vi "Teleop_Debugger_02182012.vi"(10 "Match Info":T3={"Autonomous Elapsed Seconds"=0.0, "TeleOp Elapsed Seconds"=0.0, "Disabled Elapsed Seconds"=0.0, "Visited Autonomous"=FALSE, "Visited TeleOp"=FALSE, "Visited Disabled"=FALSE, "Autonomous Settings"={"Autonomous Style"=enum."Independent", "VI Refnum"=refnum}}, 11 "Call Context":T4) -> ()   [LabVIEW 2011]
doc: "This VI is called for each TeleOp packet received from the DS where the robot is not disabled. It is often used to read from the joysticks and update I/O or to update setpoints for timed control loops. It should complete and return within 20 milliseconds or it may miss DS packets."
uses:
  <vilib>/Rock Robotics/WPI/DriverStation/WPI_DriverStationDerivedRobotMode.ctl
  <vilib>/Rock Robotics/WPI/DriverStation/WPI_DriverStationMatch Info.ctl
  <vilib>/Rock Robotics/WPI/Joystick/WPI_JoystickButtonState.ctl
  Robot Global Data.vi
  <vilib>/Rock Robotics/WPI/RobotDrive/WPI_RobotDriveArcadeDrive_Standard(NoSaturation).vi
  <vilib>/Rock Robotics/WPI/DriverStation/DriverStationLCD/WPI_DriverStationLCDLCDLine.ctl
  <vilib>/addons/control/pid/NI_PID_pid.lvlib
  <vilib>/addons/control/pid/pid.llb/PID (DBL).vi
panel:
  out "KINECT_BTNS":T1
  out "LEFT_ARM_AXES":T2
  out "RIGHT_ARM_AXES":T2
  in  "Ball_Sucker_Speed":cluster{"time":dbl, "Arm Pos 1":dbl}[](array[cluster])=[{"time"=2.2540983606557377, "Arm Pos 1"=-0.5639931736228638}] {"Arm Pos 1" scale=1.0..-1.0 scale format="%#_4g"; "time" scale=0.0..5.0}
  in  "Shoot_Feed_Speed":cluster{"time":dbl, "Arm Pos 1":dbl}[](array[cluster])=[{"time"=2.2540983606557377, "Arm Pos 1"=-0.5639931736228638}] {"Arm Pos 1" scale=1.0..-1.0 scale format="%#_4g"; "time" scale=0.0..5.0}
  in  "Shooter_Speed":cluster{"time":dbl, "Arm Pos 1":dbl}[](array[cluster])=[{"time"=2.2540983606557377, "Arm Pos 1"=-0.5639931736228638}] {"Arm Pos 1" scale=1.0..-1.0 scale format="%#_4g"; "time" scale=0.0..5.0}
  in  "REV Lift Limit":dbl(slide)=-0.7802197802197803 scale=1.0..-1.0
  in  "FWD Lift Limit":dbl(slide)=0.7252747252747253 scale=1.0..-1.0
  out "Lift PWR":dbl(slide) scale=-1.0..1.0
  in  "Down Arm Limit":dbl(knob)=0.6049517955629627 scale=1.0..-1.0 scale format="%#_4g"
  in  "UP Arm Limit":dbl(knob)=-0.5066217798191952 scale=1.0..-1.0 scale format="%#_4g"
  out "Arm PWR":dbl(knob) scale=-1.0..1.0
  in  "ShooterAngle3":cluster{"time":dbl, "Arm Pos 1":dbl}[](array[cluster])=[{"time"=2.2540983606557377, "Arm Pos 1"=-0.5639931736228638}] {"Arm Pos 1" scale=1.0..-1.0 scale format="%#_4g"; "time" scale=0.0..5.0}
  in  "ShooterAngle2":cluster{"time":dbl, "Arm Pos 1":dbl}[](array[cluster])=[{"time"=2.2540983606557377, "Arm Pos 1"=-0.5639931736228638}] {"Arm Pos 1" scale=1.0..-1.0 scale format="%#_4g"; "time" scale=0.0..5.0}
  in  "ShooterAngle1":cluster{"time":dbl, "Arm Pos 1":dbl}[](array[cluster])=[{"time"=2.2540983606557377, "Arm Pos 1"=-0.5639931736228638}] {"Arm Pos 1" scale=1.0..-1.0 scale format="%#_4g"; "time" scale=0.0..5.0}
  in  "Boost_Rate":dbl=1.5
  out "JS1_BTNS":T1
  out "JS1_AXES":T2
  out "JS2_BTNS":T1
  out "JS2_AXES":T2
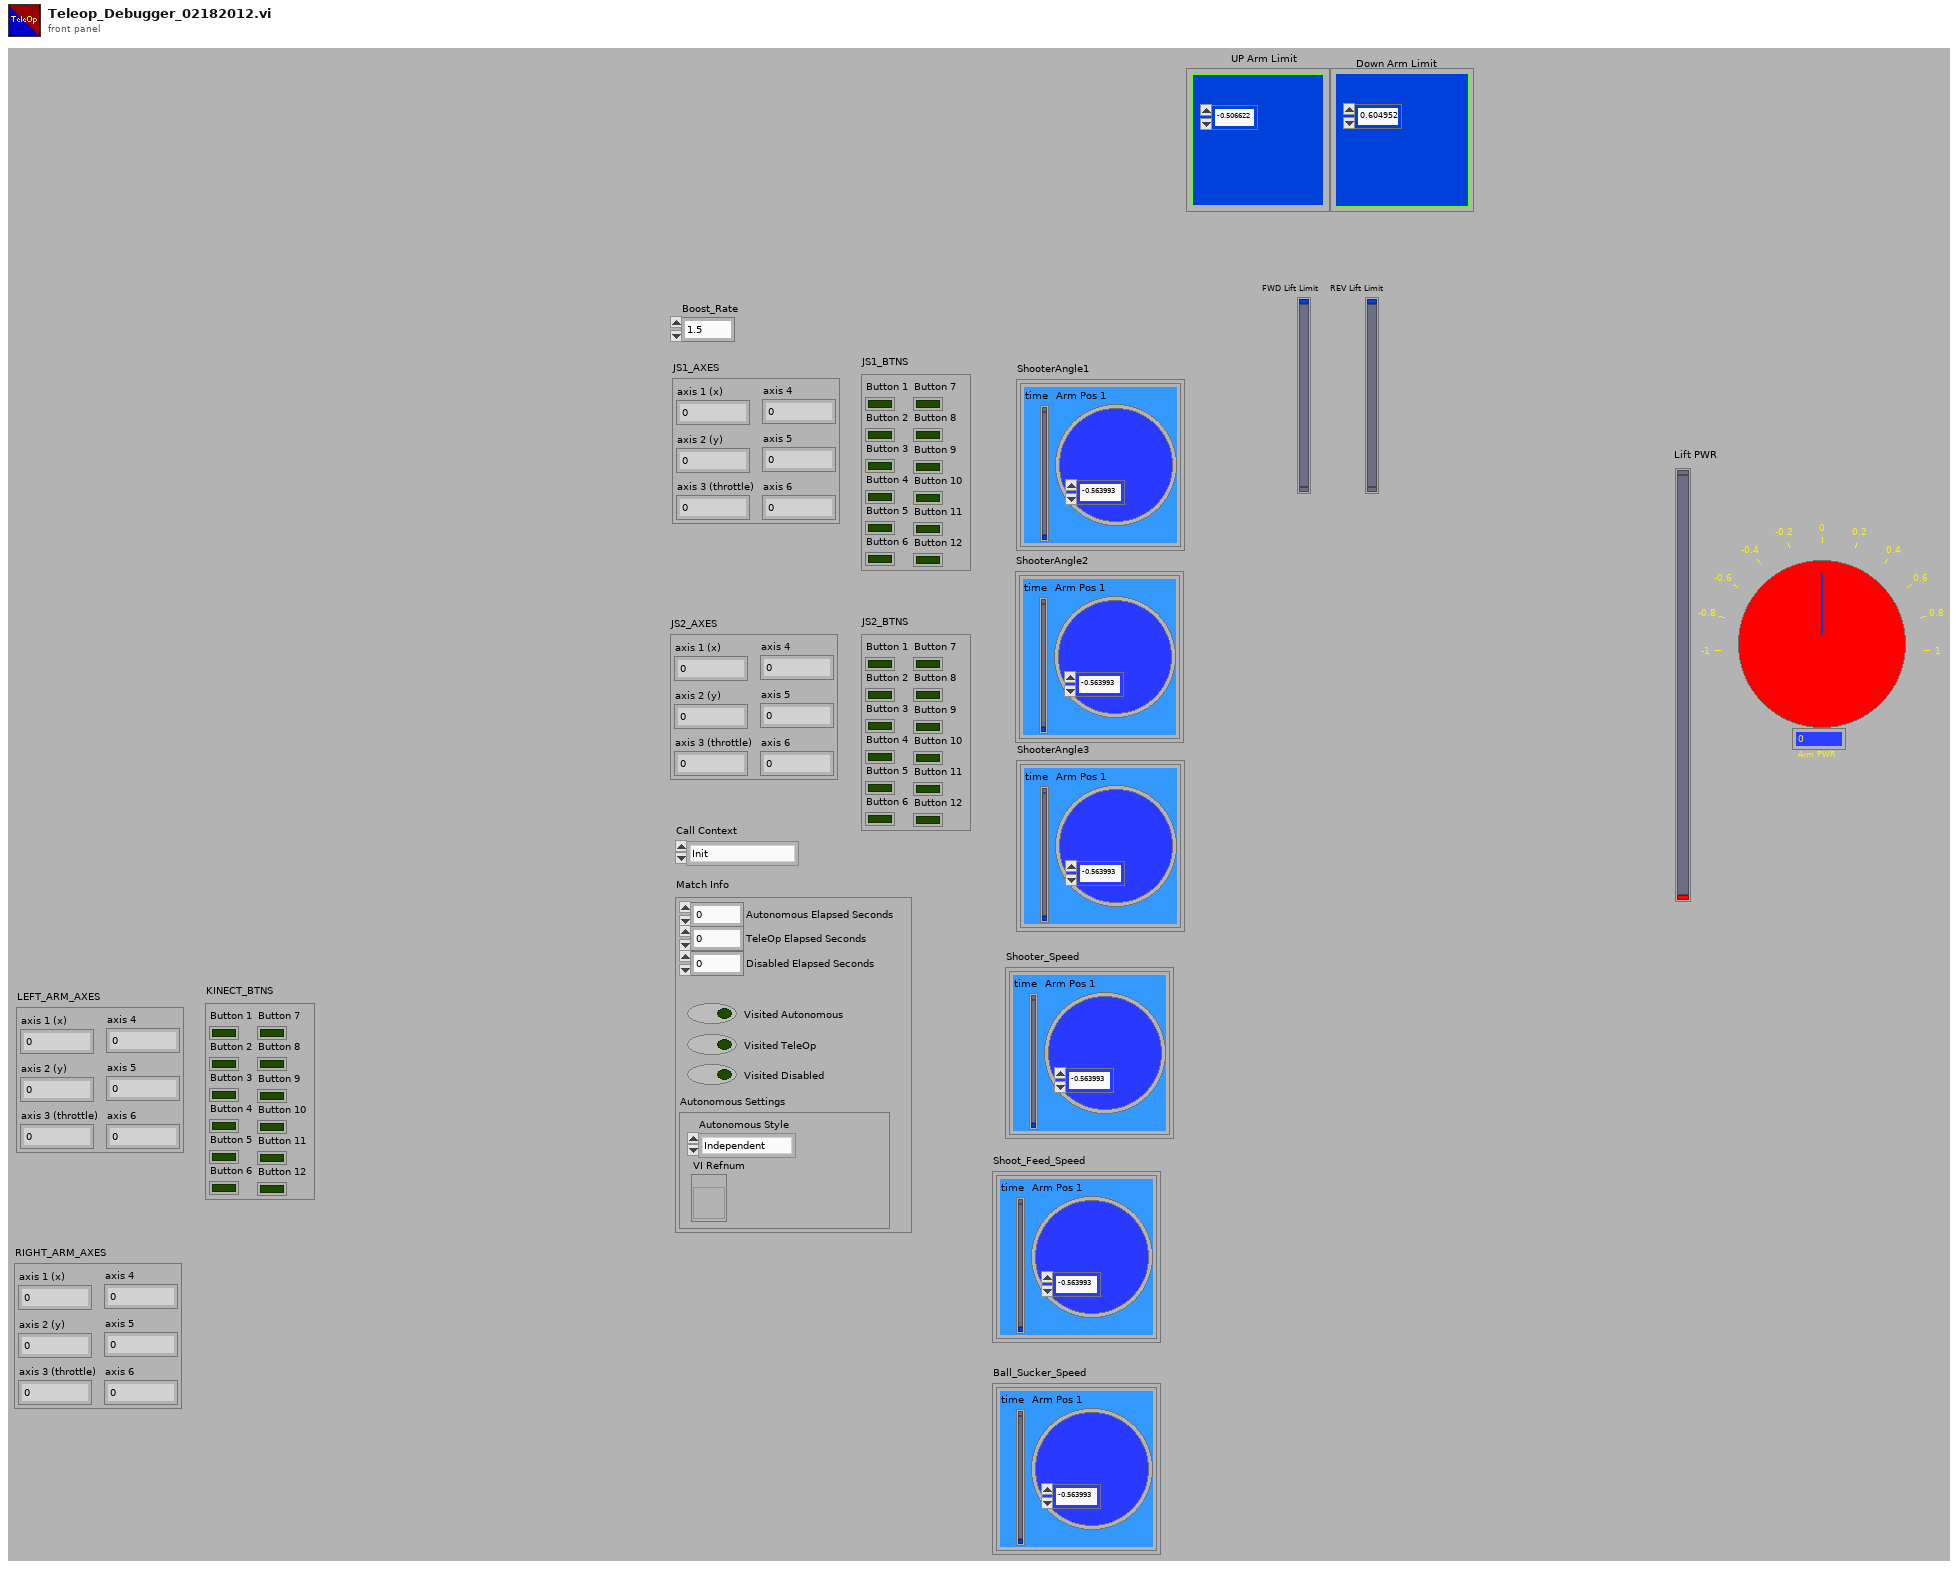
[diagram p1: front panel]
types:
  T1 = typedef "WPI_JoystickButtonState.ctl" = cluster{"Button 1":bool, "Button 2":bool, "Button 3":bool, "Button 4":bool, "Button 5":bool, "Button 6":bool, "Button 7":bool, "Button 8":bool, "Button 9":bool, "Button 10":bool, "Button 11":bool, "Button 12":bool}
  T2 = cluster{"axis 1 (x)":dbl, "axis 2 (y)":dbl, "axis 3 (throttle)":dbl, "axis 4":dbl, "axis 5":dbl, "axis 6":dbl}
  T3 = typedef "WPI_DriverStationMatch Info.ctl" = cluster{"Autonomous Elapsed Seconds":dbl, "TeleOp Elapsed Seconds":dbl, "Disabled Elapsed Seconds":dbl, "Visited Autonomous":bool, "Visited TeleOp":bool, "Visited Disabled":bool, "Autonomous Settings":cluster{"Autonomous Style":enum16{"Iterative", "Independent"}, "VI Refnum":refnum<vi>}}
  T4 = typedef "WPI_DriverStationDerivedRobotMode.ctl" = enum16{"Init", "Execute", "Stop"}
  T5 = typedef "WPI_JoystickDevRef.ctl" = cluster{"Device":T6}
  T6 = typedef "WPI_JoystickDeviceEnum.ctl" = enum16{"USB 1", "USB 2", "USB 3", "USB 4", "Kinect 1", "Kinect 2"}
  T7 = typedef "WPI_MotorControlDeviceRef.ctl" = cluster{"DeviceStatus":errorcluster, "Type":enum16{"PWM", "CAN"}, "PWM":cluster{"Digital Module":T8, "PWM Channel":T9, "DeadBand":T10}, "CAN":cluster{"Device Number":u8, "Control Mode":T11, "Semaphore":T12, "Max Vout":dbl}, "Invert":bool, "TransformRef":T13, "InvTransformRef":T13}
  T8 = typedef "FPGA_TypedefDigitalModule.ctl" = enum16{"Digital Module 1", "Digital Module 2"}
  T9 = typedef "FPGA_DIOPWMChannel.ctl" = enum8{"PWM 1", "PWM 2", "PWM 3", "PWM 4", "PWM 5", "PWM 6", "PWM 7", "PWM 8", "PWM 9", "PWM 10", "Invalid"}
  T10 = typedef "WPI_PWMDeadband.ctl" = cluster{"Name":string, "maxPositivePwm":i32, "minPositivePwm":i32, "centerPwm":i32, "maxNegativePwm":i32, "minNegativePwm":i32, "angularRange":u16}
  T11 = typedef "WPI_CANJaguar_ControlMode.ctl" = enum8{"Percent VBus", "Current", "Speed", "Position", "Voltage"}
  T12 = typedef "Semaphore RefNum" = refnum<k1>
  T13 = typedef "WPI_PWMTransform_ConPane.ctl" = refnum<vi>
  T14 = typedef "WPI_DriverStationLCDLCDLine.ctl" = enum16{"Main - Line 1", "User - Line 2", "User - Line 3", "User - Line 4", "User - Line 5", "User - Line 6"}
  T15 = typedef "WPI_ServoDeviceRef.ctl" = cluster{"DeviceStatus":errorcluster, "Digital Module":T8, "PWM Channel":T9, "DeadBand":T10}
  T16 = typedef "WPI_RobotDriveDevRef.ctl" = cluster{"DevStatus":errorcluster, "Motors[]":T7[], "Square Inputs":bool, "Max Output":dbl, "Isochronous":bool}
  T17 = cluster{"proportional gain (Kc)":dbl, "integral time (Ti, min)":dbl, "derivative time (Td, min)":dbl}
  T18 = typedef "WPI_AnalogChannelDevRef.ctl" = cluster{"DevStatus":errorcluster, "Analog Module":T19, "Analog Channel":T20}
  T19 = typedef "FPGA_TypedefAnalogModule.ctl" = enum16{"Analog Module 1", "Analog Module 2"}
  T20 = typedef "FPGA_AIChannel.ctl" = enum8{"AI 1", "AI 2", "AI 3", "AI 4", "AI 5", "AI 6", "AI 7", "AI 8", "Invalid"}
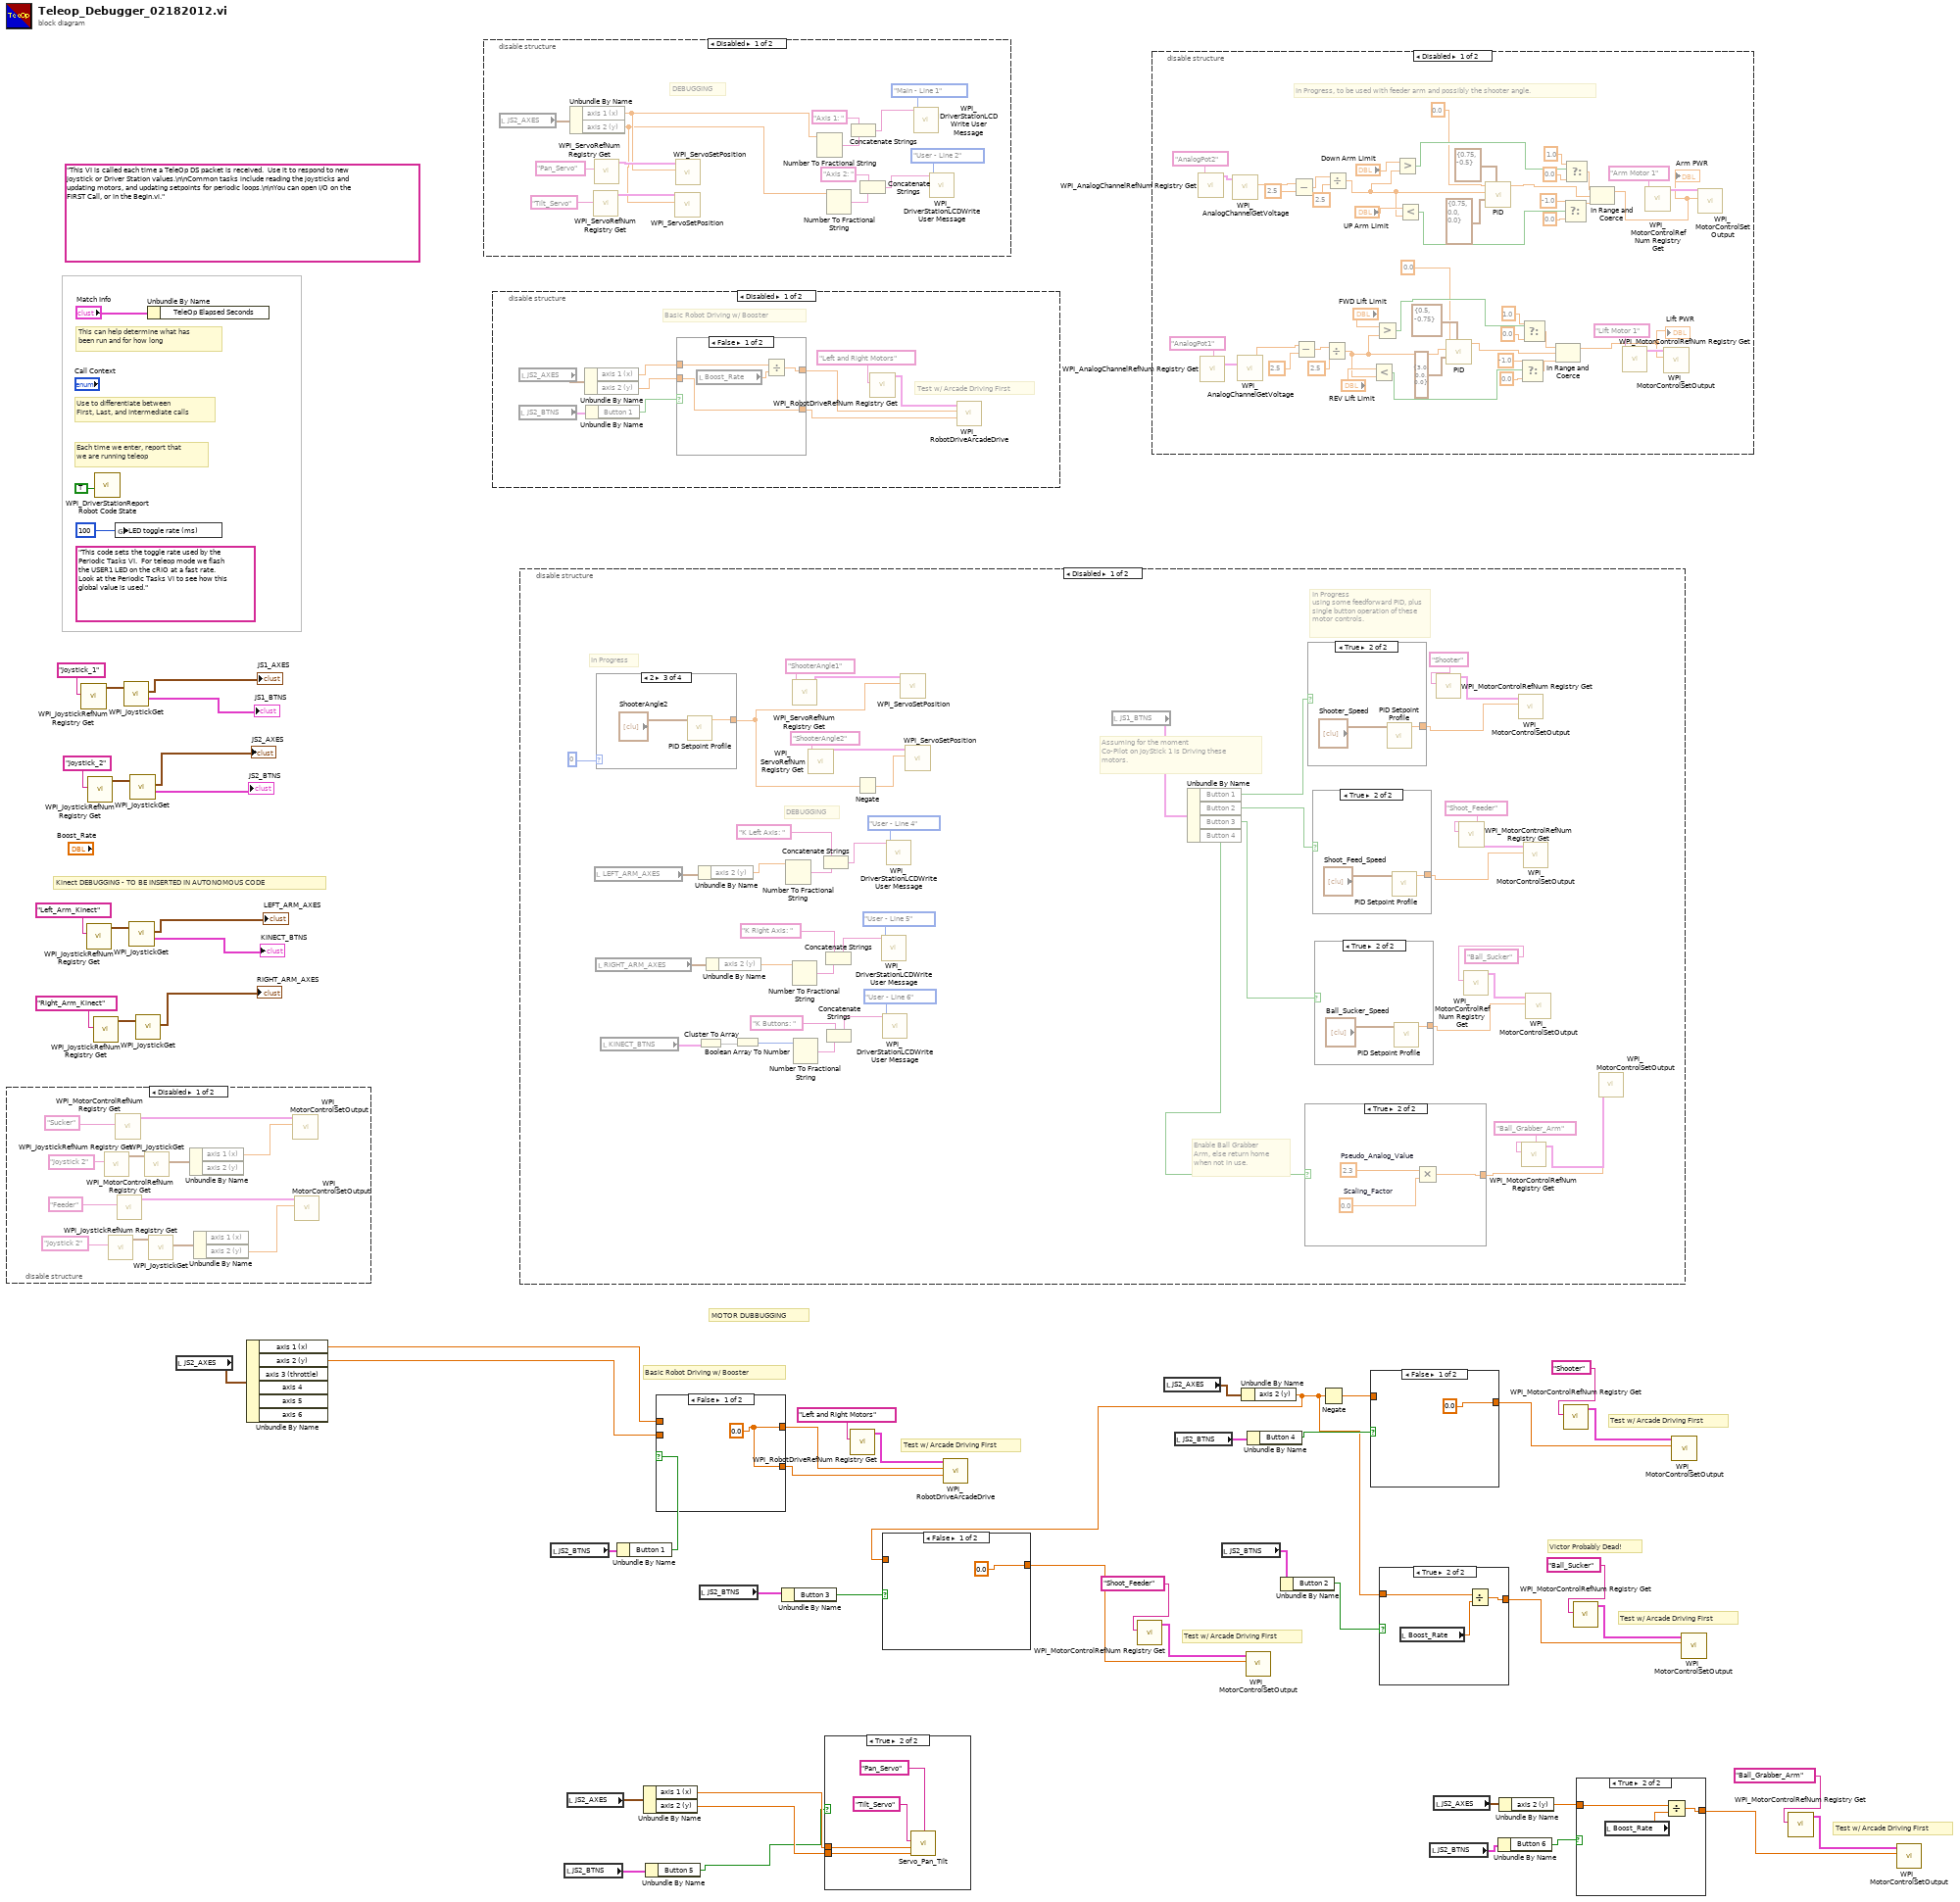
[diagram p0: block diagram]
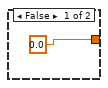
[diagram p3: hidden frame]
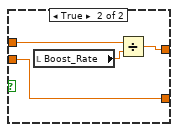
[diagram p4: hidden frame]
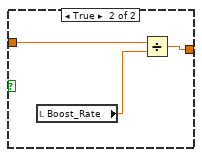
[diagram p5: hidden frame]
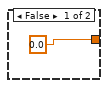
[diagram p6: hidden frame]
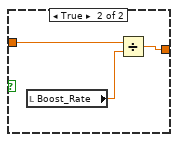
[diagram p7: hidden frame]
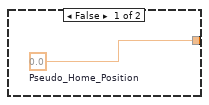
[diagram p10: hidden frame]
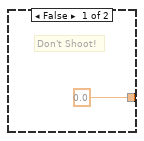
[diagram p11: hidden frame]
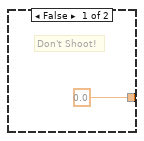
[diagram p12: hidden frame]
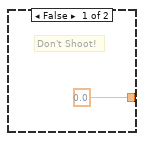
[diagram p13: hidden frame]
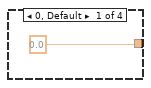
[diagram p14: hidden frame]
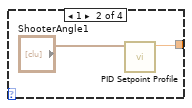
[diagram p15: hidden frame]
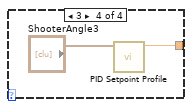
[diagram p16: hidden frame]
diagram:
  (unwired) "This code sets the toggle rate used by the Periodic Tasks VI.  For teleop mode we flash the USER1 LED on the cRIO at a fast rate.  Look at the Periodic Tasks VI to see how this global value is used."
  (unwired) "This VI is called each time a TeleOp DS packet is received.  Use it to respond to new joystick or Driver Station values.\n\nCommon tasks include reading the joysticks and updating motors, and updating setpoints for periodic loops.\n\nYou can open I/O on the FIRST Call, or in the Begin.vi."
  # "Victor Probably Dead!"
  # "Test w/ Arcade Driving First"
  # "Basic Robot Driving w/ Booster"
  # "Test w/ Arcade Driving First"
  # "Test w/ Arcade Driving First"
  # "Test w/ Arcade Driving First"
  # "Test w/ Arcade Driving First"
  # "MOTOR DUBBUGGING"
  # "Kinect DEBUGGING - TO BE INSERTED IN AUTONOMOUS CODE"
  # "Each time we enter, report that\nwe are running teleop"
  # "Use to differentiate between\nFirst, Last, and Intermediate calls"
  # "This can help determine what has\nbeen run and for how long"
  n1 = disable-structure shown="Disabled" {
    frame Disabled {
      n2 = call <vilib>:"WPI_JoystickRefNum Registry Get.vi"("refnum name"="Joystick 2") -> ("JoystickDevRef"=w67:T5)  [unwired: 1 in, 9 out]
      n3 = call <vilib>:"WPI_JoystickRefNum Registry Get.vi"("refnum name"="Joystick 2") -> ("JoystickDevRef"=w61:T5)  [unwired: 1 in, 9 out]
      n4 = call <vilib>:"WPI_MotorControlRefNum Registry Get.vi"("refnum name"="Sucker") -> ("MotorControlDevRef"=w66:T7)  [unwired: 9 in, 1 out]
      n5 = call <vilib>:"WPI_MotorControlRefNum Registry Get.vi"("refnum name"="Feeder") -> ("MotorControlDevRef"=w60:T7)  [unwired: 9 in, 1 out]
      n6 = call <vilib>:"WPI_JoystickGet.vi"("JoystickDevRef"=w67) -> ("Axes"=w69:T2)  [unwired: 1 in, 5 out]
      n7 = call <vilib>:"WPI_JoystickGet.vi"("JoystickDevRef"=w61) -> ("Axes"=w63:T2)  [unwired: 1 in, 5 out]
      n8 = Unbundle By Name(w69) -> ("axis 1 (x)"=w64:dbl)  [unwired: 1 out]
      n9 = Unbundle By Name(w63) -> ("axis 2 (y)"=w58:dbl)  [unwired: 1 out]
      n10 = call <vilib>:"WPI_MotorControlSetOutput.vi"("Output"=w64, "MotorControlDevRef"=w66) -> ()  [unwired: 8 in, 2 out]
      n11 = call <vilib>:"WPI_MotorControlSetOutput.vi"("Output"=w58, "MotorControlDevRef"=w60) -> ()  [unwired: 8 in, 2 out]
    }
    frame Enabled {
    }
  }
  n12 = call <vilib>:"WPI_JoystickRefNum Registry Get.vi"("refnum name"="Joystick_1") -> ("JoystickDevRef"=w50:T5)  [unwired: 1 in, 9 out]
  n13 = call <vilib>:"WPI_JoystickRefNum Registry Get.vi"("refnum name"="Left_Arm_Kinect") -> ("JoystickDevRef"=w43:T5)  [unwired: 1 in, 9 out]
  n14 = call <vilib>:"WPI_JoystickRefNum Registry Get.vi"("refnum name"="Joystick_2") -> ("JoystickDevRef"=w52:T5)  [unwired: 1 in, 9 out]
  n15 = call <vilib>:"WPI_JoystickRefNum Registry Get.vi"("refnum name"="Right_Arm_Kinect") -> ("JoystickDevRef"=w45:T5)  [unwired: 1 in, 9 out]
  n16 = call <vilib>:"WPI_DriverStationReport Robot Code State.vi"("TeleOp"=TRUE ("Autonomous")) -> ()  [unwired: 10 in, 1 out]
  n17 = global write "Robot Global Data.vi" "LED toggle rate (ms)"(u32 100 ("LED ms toggle rate")) -> ()
  n18 = call <vilib>:"WPI_JoystickGet.vi"("JoystickDevRef"=w50) -> ("Buttons"=→"JS1_BTNS":T1, "Axes"=→"JS1_AXES":T2)  [unwired: 1 in, 4 out]
  n19 = call <vilib>:"WPI_JoystickGet.vi"("JoystickDevRef"=w43) -> ("Buttons"=→"KINECT_BTNS":T1, "Axes"=→"LEFT_ARM_AXES":T2)  [unwired: 1 in, 4 out]
  n20 = call <vilib>:"WPI_JoystickGet.vi"("JoystickDevRef"=w52) -> ("Buttons"=→"JS2_BTNS":T1, "Axes"=→"JS2_AXES":T2)  [unwired: 1 in, 4 out]
  n21 = call <vilib>:"WPI_JoystickGet.vi"("JoystickDevRef"=w45) -> ("Axes"=→"RIGHT_ARM_AXES":T2)  [unwired: 1 in, 5 out]
  n22 = Unbundle By Name("Match Info") -> ()  [unwired: 1 out]
  n23 = local read "JS2_AXES"() -> (w25:T2)
  n24 = Unbundle By Name(w25) -> ("axis 1 (x)"=w21:dbl, "axis 2 (y)"=w20:dbl)  [unwired: 4 out]
  n25 = disable-structure shown="Disabled" {
    frame Disabled {
      # "DEBUGGING"
      n26 = local read "JS2_AXES"() -> (w70:T2)
      n27 = Unbundle By Name(w70) -> ("axis 1 (x)"=w72:dbl, "axis 2 (y)"=w71:dbl)
      n28 = call <vilib>:"WPI_ServoRefNum Registry Get.vi"("refnum name"="Tilt_Servo") -> ("ServoDeviceRef"=w83:T15)  [unwired: 9 in, 1 out]
      n29 = call <vilib>:"WPI_ServoRefNum Registry Get.vi"("refnum name"="Pan_Servo") -> ("ServoDeviceRef"=w81:T15)  [unwired: 9 in, 1 out]
      n30 = call <vilib>:"WPI_ServoSetPosition.vi"("Position"=w71, "ServoDeviceRef"=w83) -> ()  [unwired: 8 in, 2 out]
      n31 = call <vilib>:"WPI_ServoSetPosition.vi"("Position"=w72, "ServoDeviceRef"=w81) -> ()  [unwired: 8 in, 2 out]
      n32 = Number To Fractional String(number=w72) -> (F-format string=w78:string)  [unwired: 3 in]
      n33 = Number To Fractional String(number=w71) -> (F-format string=w76:string)  [unwired: 3 in]
      n34 = Concatenate Strings("Axis 1: ", w78) -> (w75:string)
      n35 = Concatenate Strings("Axis 2: ", w76) -> (w73:string)
      n36 = call <vilib>:"WPI_DriverStationLCDWrite User Message.vi"("line text"=w75, "line"=WPI_DriverStationLCDLCDLine."Main - Line 1") -> ()  [unwired: 13 in, 1 out]
      n37 = call <vilib>:"WPI_DriverStationLCDWrite User Message.vi"("line text"=w73, "line"=WPI_DriverStationLCDLCDLine."User - Line 2") -> ()  [unwired: 13 in, 1 out]
    }
    frame Enabled {
    }
  }
  n38 = disable-structure shown="Disabled" {
    frame Disabled {
      # "Basic Robot Driving w/ Booster"
      # "Test w/ Arcade Driving First"
      n39 = local read "JS2_BTNS"() -> (w90:T1)
      n40 = local read "JS2_AXES"() -> (w91:T2)
      n41 = Unbundle By Name(w91) -> ("axis 1 (x)"=w87:dbl, "axis 2 (y)"=w86:dbl)
      n42 = Unbundle By Name(w90) -> ("Button 1"=w85:bool)
      n43 = case shown="False" w85 {
        tunnel: w86 -> [w94 w98]
        tunnel: [w94 w98] -> w88
        tunnel: w87 -> [w97 w99]
        tunnel: [w96 w99] -> w89
        frame False {
          n44 = local read "Boost_Rate"() -> (w95:dbl)
          n45 = Divide(x=w97, y=w95) -> (x/y=w96:dbl)
        }
        frame True {
        }
      }
      n46 = call <vilib>:"WPI_RobotDriveRefNum Registry Get.vi"("refnum name"="Left and Right Motors") -> ("RobotDriveDevRef"=w92:T16)  [unwired: 1 in, 9 out]
      n47 = call-poly <vilib>:"WPI_RobotDriveArcadeDrive.vi"("Y axis value"=w88, "X axis value"=w89, "RobotDriveDevRef"=w92) -> ()  [unwired: 7 in, 2 out]
    }
    frame Enabled {
    }
  }
  n48 = disable-structure shown="Disabled" {
    frame Disabled {
      # "DEBUGGING"
      # "Enable Ball Grabber\nArm, else return home\nwhen not in use."
      # "Assuming for the moment\nCo-Pilot on JoyStick 1 is Driving these\nmotors."
      # "In Progress\nusing some feedforward PID, plus\nsingle button operation of these \nmotor controls."
      # "In Progress"
      n49 = local read "LEFT_ARM_AXES"() -> (w110:T2)
      n50 = local read "RIGHT_ARM_AXES"() -> (w107:T2)
      n51 = case shown="2" 0 {
        tunnel: [0.0 w157 w159 w161] -> w137
        frame 0, Default {
        }
        frame 1 {
          n52 = call <vilib>:"PID Setpoint Profile.vi"("setpoint profile"="ShooterAngle1") -> ("setpoint"=w157:dbl)  [unwired: 2 in, 6 out]
        }
        frame 2 {
          n53 = call <vilib>:"PID Setpoint Profile.vi"("setpoint profile"="ShooterAngle2") -> ("setpoint"=w159:dbl)  [unwired: 2 in, 6 out]
        }
        frame 3 {
          n54 = call <vilib>:"PID Setpoint Profile.vi"("setpoint profile"="ShooterAngle3") -> ("setpoint"=w161:dbl)  [unwired: 2 in, 6 out]
        }
      }
      n55 = local read "KINECT_BTNS"() -> (w102:T1)
      n56 = Unbundle By Name(w110) -> ("axis 2 (y)"=w109:dbl)
      n57 = Cluster To Array(cluster=w102) -> (array=w101:bool[])
      n58 = Unbundle By Name(w107) -> ("axis 2 (y)"=w108:dbl)
      n59 = Boolean Array To Number(Boolean array=w101) -> (number=w100:u32)
      n60 = Number To Fractional String(number=w109) -> (F-format string=w116:string)  [unwired: 3 in]
      n61 = call <vilib>:"WPI_ServoRefNum Registry Get.vi"("refnum name"="ShooterAngle1") -> ("ServoDeviceRef"=w141:T15)  [unwired: 1 in, 9 out]
      n62 = Number To Fractional String(number=w108) -> (F-format string=w114:string)  [unwired: 3 in]
      n63 = Number To Fractional String(number=w100) -> (F-format string=w105:string)  [unwired: 3 in]
      n64 = call <vilib>:"WPI_ServoRefNum Registry Get.vi"("refnum name"="ShooterAngle2") -> ("ServoDeviceRef"=w139:T15)  [unwired: 1 in, 9 out]
      n65 = Concatenate Strings("K Left Axis: ", w116) -> (w113:string)
      n66 = Concatenate Strings("K Right Axis: ", w114) -> (w111:string)
      n67 = Concatenate Strings("K Buttons: ", w105) -> (w103:string)
      n68 = Negate(x=w137) -> (-x=w138:dbl)
      n69 = call <vilib>:"WPI_DriverStationLCDWrite User Message.vi"("line text"=w111, "line"=WPI_DriverStationLCDLCDLine."User - Line 5") -> ()  [unwired: 13 in, 1 out]
      n70 = call <vilib>:"WPI_DriverStationLCDWrite User Message.vi"("line text"=w103, "line"=WPI_DriverStationLCDLCDLine."User - Line 6") -> ()  [unwired: 13 in, 1 out]
      n71 = call <vilib>:"WPI_DriverStationLCDWrite User Message.vi"("line text"=w113, "line"=WPI_DriverStationLCDLCDLine."User - Line 4") -> ()  [unwired: 13 in, 1 out]
      n72 = call <vilib>:"WPI_ServoSetPosition.vi"("Position"=w137, "ServoDeviceRef"=w141) -> ()  [unwired: 1 in, 9 out]
      n73 = call <vilib>:"WPI_ServoSetPosition.vi"("Position"=w138, "ServoDeviceRef"=w139) -> ()  [unwired: 1 in, 9 out]
      n74 = local read "JS1_BTNS"() -> (w126:T1)
      n75 = Unbundle By Name(w126) -> ("Button 1"=w125:bool, "Button 2"=w124:bool, "Button 3"=w123:bool, "Button 4"=w120:bool)
      n76 = case shown="True" w120 {
        tunnel: [w143 w144] -> w119
        frame False {
          w143 = 0.0  # Pseudo_Home_Position
        }
        frame True {
          w145 = 0.0  # Scaling_Factor
          w146 = 2.3  # Pseudo_Analog_Value
          n77 = Multiply(x=w146, y=w145) -> (x*y=w144:dbl)
        }
      }
      n78 = case shown="True" w125 {
        tunnel: [0.0 w154] -> w134
        frame False {
          # "Don't Shoot!"
        }
        frame True {
          n79 = call <vilib>:"PID Setpoint Profile.vi"("setpoint profile"="Shooter_Speed") -> ("setpoint"=w154:dbl)  [unwired: 2 in, 6 out]
        }
      }
      n80 = case shown="True" w124 {
        tunnel: [0.0 w151] -> w131
        frame False {
          # "Don't Shoot!"
        }
        frame True {
          n81 = call <vilib>:"PID Setpoint Profile.vi"("setpoint profile"="Shoot_Feed_Speed") -> ("setpoint"=w151:dbl)  [unwired: 2 in, 6 out]
        }
      }
      n82 = case shown="True" w123 {
        tunnel: [0.0 w148] -> w128
        frame False {
          # "Don't Shoot!"
        }
        frame True {
          n83 = call <vilib>:"PID Setpoint Profile.vi"("setpoint profile"="Ball_Sucker_Speed") -> ("setpoint"=w148:dbl)  [unwired: 2 in, 6 out]
        }
      }
      n84 = call <vilib>:"WPI_MotorControlRefNum Registry Get.vi"("refnum name"="Shooter") -> ("MotorControlDevRef"=w133:T7)  [unwired: 9 in, 1 out]
      n85 = call <vilib>:"WPI_MotorControlRefNum Registry Get.vi"("refnum name"="Shoot_Feeder") -> ("MotorControlDevRef"=w130:T7)  [unwired: 9 in, 1 out]
      n86 = call <vilib>:"WPI_MotorControlRefNum Registry Get.vi"("refnum name"="Ball_Sucker") -> ("MotorControlDevRef"=w127:T7)  [unwired: 9 in, 1 out]
      n87 = call <vilib>:"WPI_MotorControlSetOutput.vi"("Output"=w134, "MotorControlDevRef"=w133) -> ()  [unwired: 8 in, 2 out]
      n88 = call <vilib>:"WPI_MotorControlRefNum Registry Get.vi"("refnum name"="Ball_Grabber_Arm") -> ("MotorControlDevRef"=w122:T7)  [unwired: 9 in, 1 out]
      n89 = call <vilib>:"WPI_MotorControlSetOutput.vi"("Output"=w131, "MotorControlDevRef"=w130) -> ()  [unwired: 8 in, 2 out]
      n90 = call <vilib>:"WPI_MotorControlSetOutput.vi"("Output"=w128, "MotorControlDevRef"=w127) -> ()  [unwired: 8 in, 2 out]
      n91 = call <vilib>:"WPI_MotorControlSetOutput.vi"("Output"=w119, "MotorControlDevRef"=w122) -> ()  [unwired: 8 in, 2 out]
    }
    frame Enabled {
    }
  }
  n92 = local read "JS2_BTNS"() -> (w24:T1)
  n93 = local read "JS2_BTNS"() -> (w14:T1)
  n94 = local read "JS2_AXES"() -> (w13:T2)
  n95 = Unbundle By Name(w24) -> ("Button 1"=w19:bool)
  n96 = Unbundle By Name(w13) -> ("axis 1 (x)"=w3:dbl, "axis 2 (y)"=w2:dbl)
  n97 = Unbundle By Name(w14) -> ("Button 5"=w1:bool)
  n98 = case shown="False" w19 {
    tunnel: w20 -> [_ w164]
    tunnel: [w163 w164] -> w22
    tunnel: w21 -> [_ w167]
    tunnel: [w163 w166] -> w23
    frame False {
      w163 = 0.0
    }
    frame True {
      n99 = local read "Boost_Rate"() -> (w165:dbl)
      n100 = Divide(x=w167, y=w165) -> (x/y=w166:dbl)
    }
  }
  n101 = local read "JS2_BTNS"() -> (w18:T1)
  n102 = Unbundle By Name(w18) -> ("Button 3"=w17:bool)
  n103 = case shown="True" w1 {
    tunnel: w3 -> [_ w169]
    tunnel: w2 -> [_ w168]
    frame False {
    }
    frame True {
      n104 = call "Servo_Pan_Tilt.vi"("Tilt_Servo_Position"=w168, "Pan_Servo_Position"=w169, "Tilt_Servo_Name"="Tilt_Servo", "Pan_Servo_Name"="Pan_Servo") -> ()
    }
  }
  n105 = call <vilib>:"WPI_RobotDriveRefNum Registry Get.vi"("refnum name"="Left and Right Motors") -> ("RobotDriveDevRef"=w26:T16)  [unwired: 1 in, 9 out]
  n106 = call-poly <vilib>:"WPI_RobotDriveArcadeDrive.vi"("Y axis value"=w22, "X axis value"=w23, "RobotDriveDevRef"=w26) -> ()  [unwired: 7 in, 2 out]
  n107 = call <vilib>:"WPI_MotorControlRefNum Registry Get.vi"("refnum name"="Shoot_Feeder") -> ("MotorControlDevRef"=w30:T7)  [unwired: 9 in, 1 out]
  n108 = disable-structure shown="Disabled" {
    frame Disabled {
      # "In Progress, to be used with feeder arm and possibly the shooter angle."
      n109 = call <vilib>:"WPI_AnalogChannelRefNum Registry Get.vi"("refnum name"="AnalogPot2") -> ("AIDeviceRef"=w216:T18)  [unwired: 1 in, 9 out]
      n110 = call <vilib>:"WPI_AnalogChannelRefNum Registry Get.vi"("refnum name"="AnalogPot1") -> ("AIDeviceRef"=w193:T18)  [unwired: 1 in, 9 out]
      n111 = call <vilib>:"WPI_AnalogChannelGetVoltage.vi"("AIDeviceRef"=w216) -> ("Voltage"=w212:dbl)  [unwired: 1 in, 9 out]
      n112 = call <vilib>:"WPI_AnalogChannelGetVoltage.vi"("AIDeviceRef"=w193) -> ("Voltage"=w190:dbl)  [unwired: 1 in, 9 out]
      n113 = Subtract(x=w212, y=2.5) -> (x-y=w210:dbl)
      n114 = Subtract(x=w190, y=2.5) -> (x-y=w188:dbl)
      n115 = Divide(x=w188, y=2.5) -> (x/y=w176:dbl)
      n116 = Divide(x=w210, y=2.5) -> (x/y=w198:dbl)
      n117 = Less?(x="REV Lift Limit", y=w176) -> (x < y?=w185:bool)
      n118 = Greater?(x="FWD Lift Limit", y=w176) -> (0:w183:bool)
      n119 = Greater?(x="Down Arm Limit", y=w198) -> (0:w201:bool)
      n120 = Less?(x="UP Arm Limit", y=w198) -> (x < y?=w200:bool)
      n121 = call-poly <vilib>:"PID.vi"("output range"=cluster{"output high":dbl, "output low":dbl} {"output high"=0.5, "output low"=-0.75}, "PID gains"=T17 {"proportional gain (Kc)"=3.0, "integral time (Ti, min)"=0.0, "derivative time (Td, min)"=0.0}, "process variable"=w176, "setpoint"=0.0) -> ("output"=w175:dbl)  [unwired: 2 in, 5 out]
      n122 = call-poly <vilib>:"PID.vi"("output range"=cluster{"output high":dbl, "output low":dbl} {"output high"=0.75, "output low"=-0.5}, "PID gains"=T17 {"proportional gain (Kc)"=0.75, "integral time (Ti, min)"=0.0, "derivative time (Td, min)"=0.0}, "process variable"=w198, "setpoint"=0.0) -> ("output"=w199:dbl)  [unwired: 2 in, 5 out]
      n123 = Select(t=-1.0, s=w185, f=0.0) -> (s? t:f=w182:dbl)
      n124 = Select(t=1.0, s=w183, f=0.0) -> (s? t:f=w181:dbl)
      n125 = In Range and Coerce(upper limit=w181, x=w175, lower limit=w182) -> (coerced(x)=w174:dbl)  [unwired: 1 out]
      "Lift PWR" <- w174
      n126 = Select(t=-1.0, s=w200, f=0.0) -> (s? t:f=w202:dbl)
      n127 = Select(t=1.0, s=w201, f=0.0) -> (s? t:f=w203:dbl)
      n128 = In Range and Coerce(upper limit=w203, x=w199, lower limit=w202) -> (coerced(x)=w197:dbl)  [unwired: 1 out]
      "Arm PWR" <- w197
      n129 = call <vilib>:"WPI_MotorControlRefNum Registry Get.vi"("refnum name"="Lift Motor 1") -> ("MotorControlDevRef"=w195:T7)  [unwired: 1 in, 9 out]
      n130 = call <vilib>:"WPI_MotorControlRefNum Registry Get.vi"("refnum name"="Arm Motor 1") -> ("MotorControlDevRef"=w219:T7)  [unwired: 1 in, 9 out]
      n131 = call <vilib>:"WPI_MotorControlSetOutput.vi"("Output"=w174, "MotorControlDevRef"=w195) -> ()  [unwired: 3 in, 7 out]
      n132 = call <vilib>:"WPI_MotorControlSetOutput.vi"("Output"=w197, "MotorControlDevRef"=w219) -> ()  [unwired: 3 in, 7 out]
    }
    frame Enabled {
    }
  }
  n133 = local read "JS2_AXES"() -> (w39:T2)
  n134 = local read "JS2_BTNS"() -> (w38:T1)
  n135 = local read "JS2_BTNS"() -> (w16:T1)
  n136 = Unbundle By Name(w39) -> ("axis 2 (y)"=w4:dbl)
  n137 = case shown="False" w17 {
    tunnel: w4 -> [_ w223]
    tunnel: [0.0 w222] -> w29
    frame False {
    }
    frame True {
      n138 = local read "Boost_Rate"() -> (w221:dbl)
      n139 = Divide(x=w223, y=w221) -> (x/y=w222:dbl)
    }
  }
  n140 = call <vilib>:"WPI_MotorControlSetOutput.vi"("Output"=w29, "MotorControlDevRef"=w30) -> ()  [unwired: 8 in, 2 out]
  n141 = Unbundle By Name(w38) -> ("Button 4"=w37:bool)
  n142 = Unbundle By Name(w16) -> ("Button 2"=w15:bool)
  n143 = Negate(x=w4) -> (-x=w5:dbl)
  n144 = case shown="False" w37 {
    tunnel: w5 -> [_ w227]
    tunnel: [0.0 w226] -> w35
    frame False {
    }
    frame True {
      n145 = local read "Boost_Rate"() -> (w225:dbl)
      n146 = Divide(x=w227, y=w225) -> (x/y=w226:dbl)
    }
  }
  n147 = case shown="True" w15 {
    tunnel: w4 -> [_ w231]
    tunnel: [0.0 w230] -> w32
    frame False {
    }
    frame True {
      n148 = local read "Boost_Rate"() -> (w229:dbl)
      n149 = Divide(x=w231, y=w229) -> (x/y=w230:dbl)
    }
  }
  n150 = local read "JS2_BTNS"() -> (w8:T1)
  n151 = local read "JS2_AXES"() -> (w9:T2)
  n152 = Unbundle By Name(w8) -> ("Button 6"=w7:bool)
  n153 = Unbundle By Name(w9) -> ("axis 2 (y)"=w6:dbl)
  n154 = call <vilib>:"WPI_MotorControlRefNum Registry Get.vi"("refnum name"="Shooter") -> ("MotorControlDevRef"=w36:T7)  [unwired: 9 in, 1 out]
  n155 = call <vilib>:"WPI_MotorControlRefNum Registry Get.vi"("refnum name"="Ball_Sucker") -> ("MotorControlDevRef"=w33:T7)  [unwired: 9 in, 1 out]
  n156 = case shown="True" w7 {
    tunnel: w6 -> [_ w235]
    tunnel: [0.0 w234] -> w10
    frame False {
    }
    frame True {
      n157 = local read "Boost_Rate"() -> (w233:dbl)
      n158 = Divide(x=w235, y=w233) -> (x/y=w234:dbl)
    }
  }
  n159 = call <vilib>:"WPI_MotorControlSetOutput.vi"("Output"=w35, "MotorControlDevRef"=w36) -> ()  [unwired: 8 in, 2 out]
  n160 = call <vilib>:"WPI_MotorControlSetOutput.vi"("Output"=w32, "MotorControlDevRef"=w33) -> ()  [unwired: 8 in, 2 out]
  n161 = call <vilib>:"WPI_MotorControlRefNum Registry Get.vi"("refnum name"="Ball_Grabber_Arm") -> ("MotorControlDevRef"=w12:T7)  [unwired: 9 in, 1 out]
  n162 = call <vilib>:"WPI_MotorControlSetOutput.vi"("Output"=w10, "MotorControlDevRef"=w12) -> ()  [unwired: 8 in, 2 out]
